vi "Retrieve Pending IMatch Responses.vi"(8 "error in":errorcluster, 10 "Response Matcher Enq":refnum<class "Message Enqueuer.lvclass">) -> (0 "error out":errorcluster, 1 "Pending IMatch Responses":refnum<data-value>)   [LabVIEW 2024]
uses:
  Node Guard.lvclass/Node Guard.ctl
  <vilib>/ActorFramework/Specialty Messages/Reply Msg/Reply Msg.lvclass
  Response Matcher Messages/Get Pending IMatch Responses Msg/Get Pending IMatch Responses Reply Msg.lvclass
  IResponse/IMatch Response.lvclass
  <vilib>/ActorFramework/Message Enqueuer/Message Enqueuer.lvclass
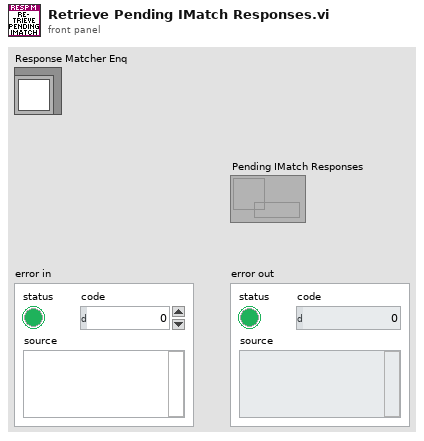
[diagram p1: front panel]
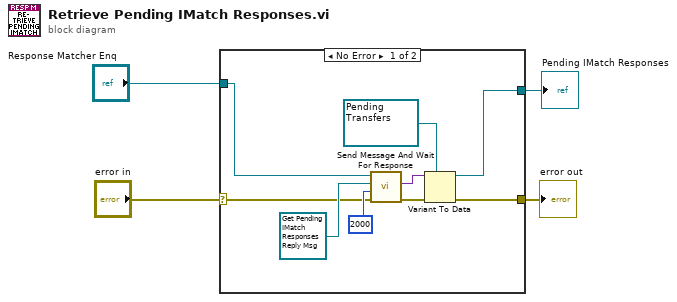
[diagram p0: block diagram]
diagram:
  n1 = case shown="No Error" "error in" {
    selector: "error in" -> [w8 w14]
    tunnel: [w7 w14] -> w3
    tunnel: "Response Matcher Enq" -> [w6 _]
    tunnel: [w5 _] -> w1
    frame No Error {
      n2 = call <vilib>:"Send Message And Wait For Response.vi"("error in (no error)"=w8, "timeout in ms (-1)"=2000, "Original Message"=refnum<class "Get Pending IMatch Responses Reply Msg.lvclass"> refnum ("CANopen.lvlib:Response Matcher.lvlib:Get Pending IMatch Responses Reply Msg.lvclass"), "Message Enqueuer in"=w6) -> ("error out"=w11:errorcluster, "Reply"=w10:variant)  [unwired: 4 in, 2 out]
      n3 = Variant To Data(error in=w11, type=refnum<data-value> refnum ("Pending IMatch Responses"), Variant=w10) -> (data=w5:refnum<data-value>, error out=w7:errorcluster)
    }
    frame Error {
    }
  }
  "error out" <- w3
  "Pending IMatch Responses" <- w1
